vi "EX1.vi"() -> ()   [LabVIEW 2024]
uses:
  <vilib>/Instr/_visa.llb/VISA Open Access Mode.ctl
  <vilib>/Instr/_visa.llb/VISA Configure Serial Port (Instr).vi
panel:
  out "etat":string
  in  "Sortie":bool
  out "sortie":string
  out "temps sortie":string
  in  "Entrer":bool
  out "entree":string
  out "temps entree":string
  in  "stop":bool
  in  "VISA resource name":refnum<visa-resource-name>
  # "TP N°5"
  # "Mekni Marwen 2ème Année Génie Electrique"
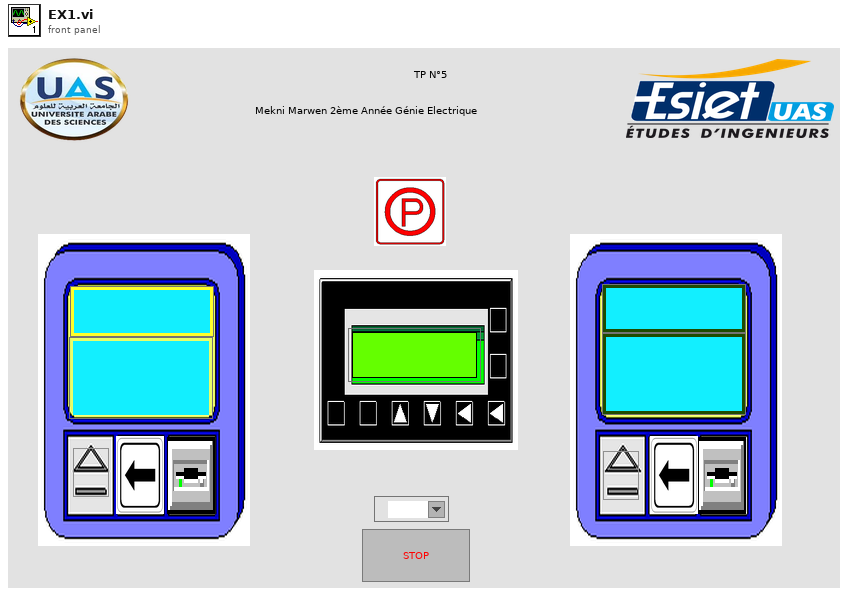
[diagram p1: front panel]
types:
  T1 = typedef "VISA Open Access Mode.ctl" = u32
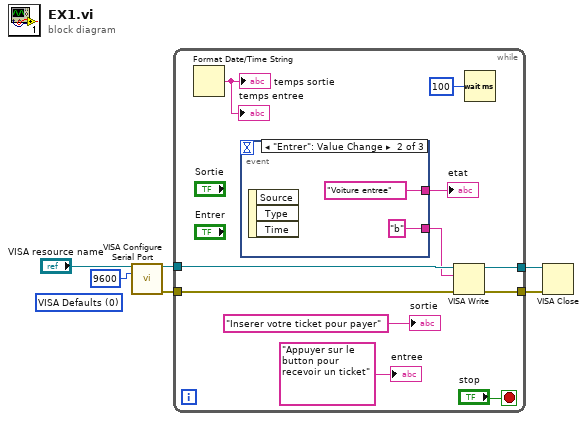
[diagram p0: block diagram]
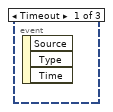
[diagram p2: hidden frame]
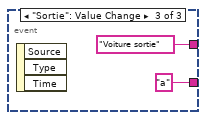
[diagram p3: hidden frame]
diagram:
  (unwired) T1 0 items=["VISA Defaults"=0, "Exclusive Lock"=1, "Load Configured Settings"=4] ("Access Mode")
  n1 = call-poly "VISA Configure Serial Port"("VISA resource name"="VISA resource name", "baud rate (9600)"=u32 9600) -> ("VISA resource name out"=w6:refnum<visa-resource-name>, "error out"=w3:errorcluster)  [unwired: 12 in]
  n2 = while {
    tunnel: w6 -> [w17]
    tunnel: [w16] -> w5
    tunnel: [w15] -> w4
    tunnel: w3 -> [w14]
    stop <- "stop" stop-if-true
    n3 = Format Date/Time String() -> (date/time string=→"temps sortie" →"temps entree":string)  [unwired: 3 in]
    n4 = event shown="[1] \"Entrer\": Value Change" {
      selector: _ -> [_ _ _]
      dyn-events: _ -> [_ _ _]
      timeout: _ -> [_ _ _]
      tunnel: [_ "b" "a"] -> w9
      tunnel: [_ "Voiture entree" "Voiture sortie"] -> w8
      event Timeout {
        n5 = event-data() -> ()  [unwired: 1 in, 3 out]
      }
      event "Entrer": Value Change {
        n6 = event-data() -> ()  [unwired: 1 in, 3 out]
      }
      event "Sortie": Value Change {
        n7 = event-data() -> ()  [unwired: 1 in, 3 out]
      }
    }
    "etat" <- w8
    n8 = VISA Write(VISA resource name=w17, write buffer=w9, error in (no error)=w14) -> (VISA resource name out=w16:refnum<visa-resource-name>, error out=w15:errorcluster)  [unwired: 1 out]
    n9 = Wait (ms)(milliseconds to wait=u32 100) -> ()  [unwired: 1 out]
    "entree" <- "Appuyer sur le button pour recevoir un ticket" ("String 3")
    "sortie" <- "Inserer votre ticket pour payer" ("String 4")
  }
  n10 = VISA Close(VISA resource name=w5, error in (no error)=w4) -> ()  [unwired: 1 out]
